vi "Get File.vi"(7 "output file path":path=path "", 8 "error in (no error)":errorcluster, 10 "id":u32, 11 "eLab in":refnum<class "PL eLabFTW Client.lvclass">) -> (0 "error out":errorcluster, 2 "data":string, 3 "eLab out":refnum<class "PL eLabFTW Client.lvclass">)   [LabVIEW 2015, in "PL eLabFTW Client.lvclass"]
doc: "Gets file with the specified id."
uses:
  PL eLabFTW Client.lvclass
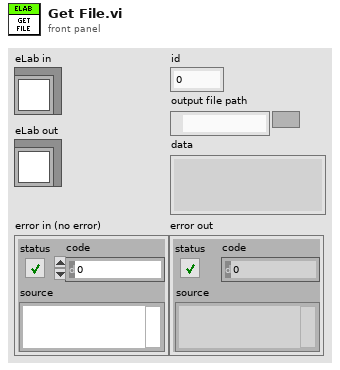
[diagram p1: front panel]
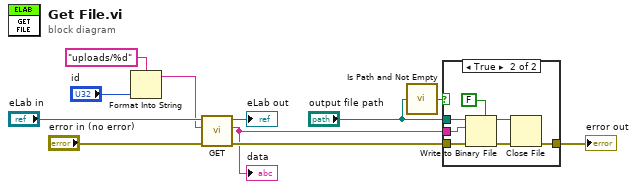
[diagram p0: block diagram]
diagram:
  n1 = Format Into String(format string="uploads/%d", "id") -> (resulting string=w7:string)  [unwired: 2 in, 1 out]
  n2 = call "GET.vi"("error in (no error)"="error in (no error)", "relative URL"=w7, "eLab in"="eLab in") -> ("error out"=w5:errorcluster, "response body"=w1:string, "eLab out"=→"eLab out":refnum<class "PL eLabFTW Client.lvclass">)  [unwired: 6 in]
  "data" <- w1
  n3 = call <vilib>:"Is Path and Not Empty.vi"("path"="output file path") -> ("Is Path and Not Empty?"=w2:bool)  [unwired: 4 in]
  n4 = case shown="True" w2 {
    tunnel: w5 -> [w12 w19]
    tunnel: [w12 w15] -> w4
    tunnel: "output file path" -> [_ w18]
    tunnel: w1 -> [_ w13]
    frame False {
    }
    frame True {
      n5 = Write to Binary File(file (use dialog)=w18, data=w13, error in=w19, 5:FALSE ("prepend array or string size? (T)")) -> (refnum out=w16:refnum<file>, error out=w17:errorcluster)  [unwired: 2 in, 1 out]
      n6 = Close File(refnum=w16, error in=w17) -> (error out=w15:errorcluster)  [unwired: 1 out]
    }
  }
  "error out" <- w4
